vi "Convert Excel to NI Cluster.vi"(8 "error in":errorcluster, 11 "path":path=path "C:/Users/Blueuser/Desktop/Testing/SampleConfiguration.xlsx") -> (0 "error out":errorcluster, 3 "Chassis Settings":T18 {"Chassis Settings"."Master Chassis"."startTriggerLine" items=["None", "PFI_0", "PFI_1", "PFI_2", "PFI_3", "PFI_4", "PFI_5", "PFI_6", "PFI_7", "PFI_8", "PFI_9", "PFI_10", "PFI_11", "PFI_12", "PFI_13", "PFI_14", "PFI_15", "RTSI_PXI_TRIG_0", "RTSI_PXI_TRIG_1", "RTSI_PXI_TRIG_2", "RTSI_PXI_TRIG_3", "RTSI_PXI_TRIG_4", "RTSI_PXI_TRIG_5", "RTSI_PXI_TRIG_6", "RTSI_PXI_TRIG_7"]; "Chassis Settings"."Master Chassis"."startTrigger" items=["aiStartTrigger", "aoStartTrigger"]; "Chassis Settings"."Master Chassis"."triggerSlope" items=["Falling"=10171, "Rising"=10280]; "Chassis Settings"."Master Chassis"."triggerLine" items=["None", "PFI_0", "PFI_1", "PFI_2", "PFI_3", "PFI_4", "PFI_5", "PFI_6", "PFI_7", "PFI_8", "PFI_9", "PFI_10", "PFI_11", "PFI_12", "PFI_13", "PFI_14", "PFI_15", "RTSI_PXI_TRIG_0", "RTSI_PXI_TRIG_1", "RTSI_PXI_TRIG_2", "RTSI_PXI_TRIG_3", "RTSI_PXI_TRIG_4", "RTSI_PXI_TRIG_5", "RTSI_PXI_TRIG_6", "RTSI_PXI_TRIG_7"]; "Chassis Settings"."Master Chassis"."exportClkToLine" items=["Default_RTSI_PXI_TRIG_0", "PFI_0", "PFI_1", "PFI_2", "PFI_3", "PFI_4", "PFI_5", "PFI_6", "PFI_7", "PFI_8", "PFI_9", "PFI_10", "PFI_11", "PFI_12", "PFI_13", "PFI_14", "PFI_15", "RTSI_PXI_TRIG_0", "RTSI_PXI_TRIG_1", "RTSI_PXI_TRIG_2", "RTSI_PXI_TRIG_3", "RTSI_PXI_TRIG_4", "RTSI_PXI_TRIG_5", "RTSI_PXI_TRIG_6", "RTSI_PXI_TRIG_7"]; "Chassis Settings"."Master Chassis"."exportClk" items=["aiSampleClock", "aoSampleClock"]; "Chassis Settings"."Master Chassis"."activeEdge" items=["Falling"=10171, "Rising"=10280]; "Chassis Settings"."Master Chassis"."clkSrc" items=["Onboard10MHzClock", "PFI_0", "PFI_1", "PFI_2", "PFI_3", "PFI_4", "PFI_5", "PFI_6", "PFI_7", "PFI_8", "PFI_9", "PFI_10", "PFI_11", "PFI_12", "PFI_13", "PFI_14", "PFI_15", "RTSI_PXI_TRIG_0", "RTSI_PXI_TRIG_1", "RTSI_PXI_TRIG_2", "RTSI_PXI_TRIG_3", "RTSI_PXI_TRIG_4", "RTSI_PXI_TRIG_5", "RTSI_PXI_TRIG_6", "RTSI_PXI_TRIG_7"]; "DAQ Boards"."Counter Settings"."Position Measurements"."ZIndexMode" items=["AHighBHigh"=10040, "AHighBLow"=10041, "ALowBHigh"=10042, "ALowBLow"=10043]; "DAQ Boards"."Counter Settings"."Position Measurements"."Decoding" items=["Decoding1X"=10090, "Decoding2X"=10091, "Decoding4X"=10092, "DecodingPulseCounting"=10313]; "DAQ Boards"."Counter Settings"."Count Measurements"."CountDirection" items=["Down"=10124, "Up"=10128, "ExternallyControlled"=10326]; "DAQ Boards"."Counter Settings"."Count Measurements"."Edge" items=["Falling"=10171, "Rising"=10280]; "DAQ Boards"."Counter Settings"."Period Measurements"."Edge" items=["Falling"=10171, "Rising"=10280]; "DAQ Boards"."Counter Settings"."Frequency Measurements"."Edge" items=["Falling"=10171, "Rising"=10280]; "DAQ Boards"."Analog Outputs"."ChannelType" items=["Voltage", "Current"]; "DAQ Boards"."Analog Inputs"."ChannelType" items=["Voltage", "Current"]; "DAQ Boards"."DAQConversionRateOption" items=["Default", "Maximum"]; "DAQ Boards"."InputConfiguration" items=["NRSE"=10078, "RSE"=10083, "Differential"=10106, "Pseudodifferential"=12529, "Default"=-1]; "CAN Boards"."Log Files"."Operation" items=["ContinueLoggingInNewFile", "StopLogging"]; "CAN Boards"."Log Files"."LimitType" items=["Footprint", "Time"]; "CAN Boards"."Log Files"."TriggerType" items=["StartLoggingOnNonZero", "StartLoggingOnZero", "EnableLoggingWhenTriggerIsZero", "EnableLoggingWhenTriggerIsNonZero"]; "CAN Boards"."Log Files"."Filter" items=["LogEntireBusTraffic", "ExcludeFrameIDs", "IncludeFrameIDs"]; "CAN Boards"."Log Files"."DataLoggingFileType" items=["TDMS", "NCL"]; "CAN Boards"."TransmitOrderType" items=["AsSubmitted", "ByIdentifier"]; "CAN Boards"."TransceiverType" items=["HS", "LS", "SW"]; "CAN Boards"."Termination" items=["Off", "On"]; "CAN Boards"."Outgoing Frames"."Phase" items=["Unchanged", "Reset"]; "CAN Boards"."Outgoing Frames"."TriggerType" items=["ChannelValueChange", "TriggerChannelNotZero", "ChannelValueChangeOrTriggerChannelNotZero"]})   [LabVIEW 2019, in "Simple SysDef API.lvlib"]
uses:
  <userlib>/SimpleSysDef/Simple SysDef API.lvlib
  <userlib>/SimpleSysDef/_SubVIs/Edit Chassis_Settings.ctl
  <userlib>/SimpleSysDef/_SubVIs/Add Chassis_DAQ Master Settings.ctl
  <userlib>/SimpleSysDef/_SubVIs/Add Chassis_Type.ctl
  <userlib>/SimpleSysDef/_SubVIs/Add DAQ Hardware_Settings.ctl
  <userlib>/SimpleSysDef/_SubVIs/Add DAQ Hardware_Analog Settings.ctl
  <userlib>/SimpleSysDef/_SubVIs/Add DAQ Hardware_Digital Port Settings.ctl
  <userlib>/SimpleSysDef/_SubVIs/Add DAQ Hardware_Digital Settings.ctl
  <userlib>/SimpleSysDef/_SubVIs/Add Frequency Measurement Channels_Settings.ctl
  <userlib>/SimpleSysDef/_SubVIs/Add Count Measurement Channels_Settings.ctl
  NationalInstruments.VeriStand.SystemDefinitionAPI
  <userlib>/SimpleSysDef/_SubVIs/Add Position Measurement Channels_Settings.ctl
  <userlib>/SimpleSysDef/_SubVIs/Add FPGA Hardware_Settings.ctl
  <userlib>/SimpleSysDef/_SubVIs/Add NI-XNET CAN Hardware_Port Settings.ctl
  <userlib>/SimpleSysDef/_SubVIs/Add NI-XNET CAN Hardware_Periodic Frame Settings.ctl
  <userlib>/SimpleSysDef/_SubVIs/Add NI-XNET CAN Hardware_Frame Settings.ctl
  <userlib>/SimpleSysDef/_SubVIs/Add NI-XNET CAN Hardware_Signal Settings.ctl
  <userlib>/SimpleSysDef/_SubVIs/Add NI-XNET CAN Hardware_Sporadic Frame Settings.ctl
  <userlib>/SimpleSysDef/_SubVIs/Add NI-XNET CAN Hardware_Add Log File_Settings.ctl
  <vilib>/Utility/error.llb/Trim Whitespace One-Sided.vi
  <vilib>/regexp/Match Regular Expression.xnode
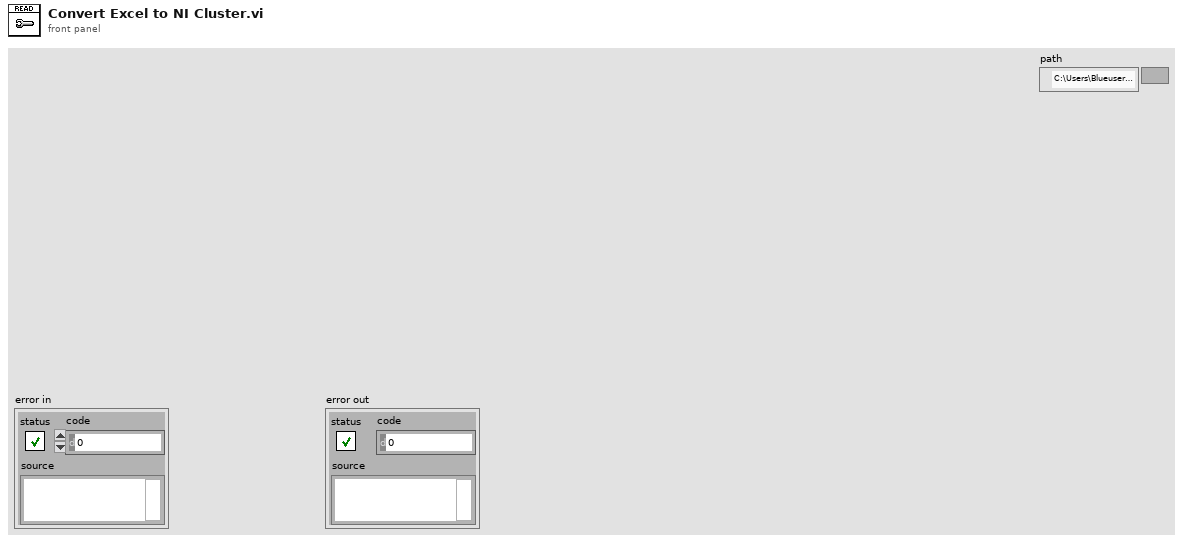
[diagram p1: front panel]
types:
  T1 = typedef "Simple SysDef API.lvlib/Edit Chassis_Settings.ctl" = cluster{"Name":string, "Master Chassis":T2}
  T2 = typedef "Simple SysDef API.lvlib/Add Chassis_DAQ Master Settings.ctl" = cluster{"Type":T3, "DAQ Name":string, "clkSrc":i32, "activeEdge":i32, "exportClk":i32, "exportClkToLine":i32, "triggerLine":i32, "triggerSlope":i32, "startTrigger":i32, "startTriggerLine":i32}
  T3 = typedef "Simple SysDef API.lvlib/Add Chassis_Type.ctl" = enum16{"None", "DAQ", "FPGA", "Timing and Sync", "Automatic"}
  T4 = typedef "Simple SysDef API.lvlib/Add DAQ Hardware_Settings.ctl" = cluster{"Name":string, "Description":string, "InputConfiguration":i32, "TurnOffHWTimedSinglePointAI":bool, "TurnOffHWTimedSinglePointAO":bool, "DAQConversionRateOption":i32, "PortWidth":u16, "Analog Inputs":T5[], "Analog Outputs":T5[], "DIO Port Settings":T6[], "Counter Settings":cluster{"Frequency Measurements":T8[], "Period Measurements":T8[], "Count Measurements":T9[], "Position Measurements":T10[]}}
  T5 = typedef "Simple SysDef API.lvlib/Add DAQ Hardware_Analog Settings.ctl" = cluster{"Name":string, "Units":string, "InitialValue":dbl, "HighLevel":dbl, "LowLevel":dbl, "Channel":u32, "ChannelType":i32, "Alias Name":string}
  T6 = typedef "Simple SysDef API.lvlib/Add DAQ Hardware_Digital Port Settings.ctl" = cluster{"portNumber":u32, "Inverted":bool, "Digital Inputs":T7[], "Digital Outputs":T7[]}
  T7 = typedef "Simple SysDef API.lvlib/Add DAQ Hardware_Digital Settings.ctl" = cluster{"Name":string, "InitialValue":bool, "DigitalLine":u32, "Alias Name":string}
  T8 = typedef "Simple SysDef API.lvlib/Add Frequency Measurement Channels_Settings.ctl" = cluster{"Name":string, "Description":string, "Units":string, "Counter":u32, "DefaultValue":dbl, "Maximum":dbl, "Minimum":dbl, "Edge":i32, "Alias Name":string}
  T9 = typedef "Simple SysDef API.lvlib/Add Count Measurement Channels_Settings.ctl" = cluster{"Name":string, "Description":string, "Units":string, "Counter":u32, "DefaultValue":dbl, "CountDirection":i32, "Edge":i32, "ResetVariable":refnum<k24>, "Alias Name":string}
  T10 = typedef "Simple SysDef API.lvlib/Add Position Measurement Channels_Settings.ctl" = cluster{"Name":string, "Description":string, "Units":string, "Counter":u32, "DefaultValue":dbl, "Decoding":i32, "ZIndexMode":i32, "Alias Name":string}
  T11 = typedef "Simple SysDef API.lvlib/Add FPGA Hardware_Settings.ctl" = cluster{"Path":path, "RIO Name":string, "Aliases":cluster{"Relative Node Path":string, "Alias Name":string}[]}
  T12 = typedef "Simple SysDef API.lvlib/Add NI-XNET CAN Hardware_Port Settings.ctl" = cluster{"Name":string, "Database Name":string, "PortNumber":u16, "ClusterName":string, "BaudRate":u32, "InlineIncoming":bool, "IncomingRate":u32, "InlineOutgoing":bool, "OutgoingRate":u32, "Termination":i32, "Echo":bool, "InputStreamQueueSize":u32, "CANBusOff":bool, "CANBusOffRate":u32, "TransceiverType":i32, "TransmitOrderType":i32, "Cyclic Frames":T13[], "Outgoing Frames":T16[], "Incoming Frames":T14[], "Log Files":T17[]}
  T13 = typedef "Simple SysDef API.lvlib/Add NI-XNET CAN Hardware_Periodic Frame Settings.ctl" = cluster{"Frame Settings":T14, "Trigger Node Path":string, "TriggerType":i32, "Disable Node Path":string}
  T14 = typedef "Simple SysDef API.lvlib/Add NI-XNET CAN Hardware_Frame Settings.ctl" = cluster{"Name":string, "ID":u32, "PayloadLength":u32, "StartTimeOffset":dbl, "Enable64Bit":bool, "Signals":T15[]}
  T15 = typedef "Simple SysDef API.lvlib/Add NI-XNET CAN Hardware_Signal Settings.ctl" = cluster{"Name":string, "Description":string, "Units":string, "DefaultValue":dbl, "Alias Name":string}
  T16 = typedef "Simple SysDef API.lvlib/Add NI-XNET CAN Hardware_Sporadic Frame Settings.ctl" = cluster{"Frame Settings":T14, "Trigger Node Path":string, "TriggerType":i32, "Disable Node Path":string, "EnableSoftwareCyclicTrigger":bool, "TransmitTime":dbl, "Phase":i32}
  T17 = typedef "Simple SysDef API.lvlib/Add NI-XNET CAN Hardware_Add Log File_Settings.ctl" = cluster{"Name":string, "Filename":string, "Destination Folder":path, "NumberOfBytesToRead":u32, "DataLoggingFileType":i32, "TDMSGroupName":string, "TDMSChannelName":string, "Filter":i32, "FrameIDs":string[], "TriggerType":i32, "LimitType":i32, "LimitValue":u32, "Operation":i32, "Retriggerable":bool, "Trigger Node Path":string}
  T18 = cluster{"Chassis Settings":T1, "DAQ Boards":T4[], "FPGA Boards":T11[], "CAN Boards":T12[]}
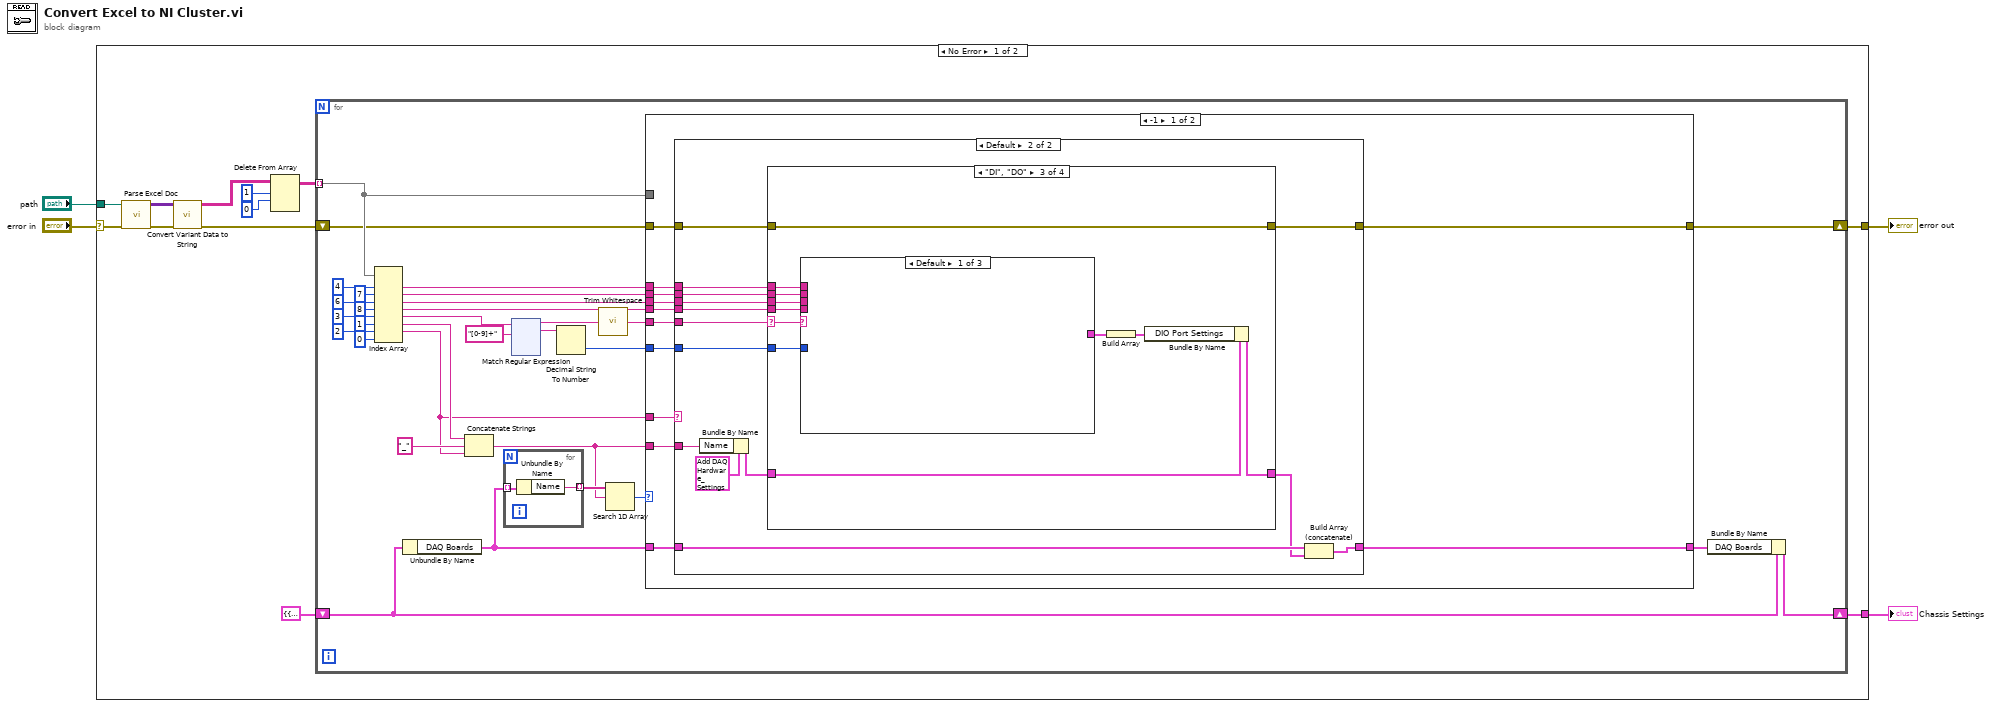
[diagram p0: block diagram]
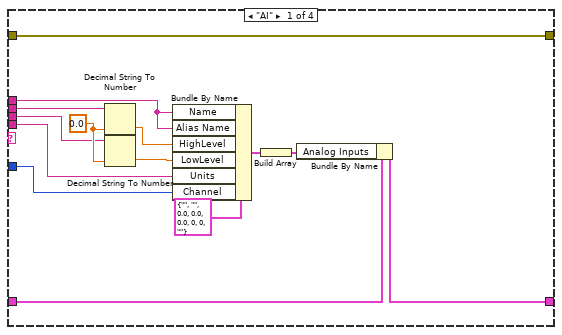
[diagram p3: hidden frame]
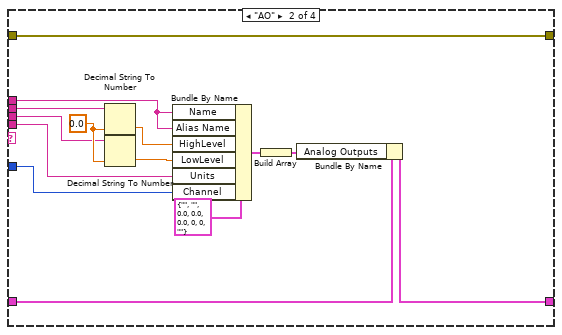
[diagram p4: hidden frame]
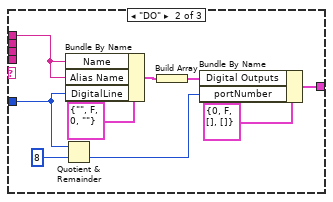
[diagram p5: hidden frame]
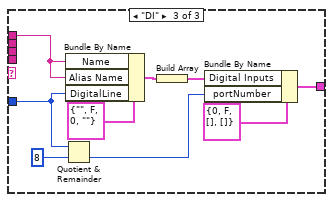
[diagram p6: hidden frame]
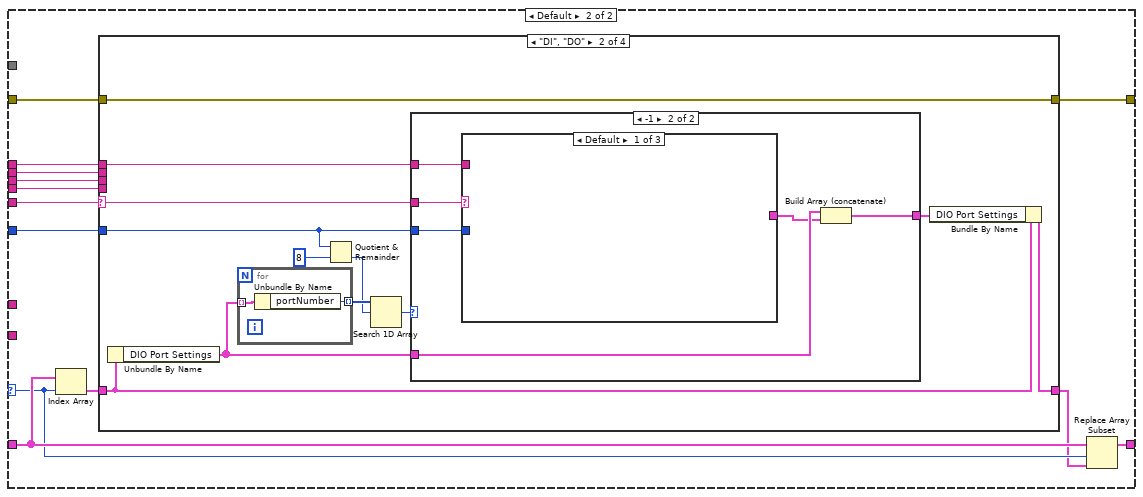
[diagram p8: hidden frame]
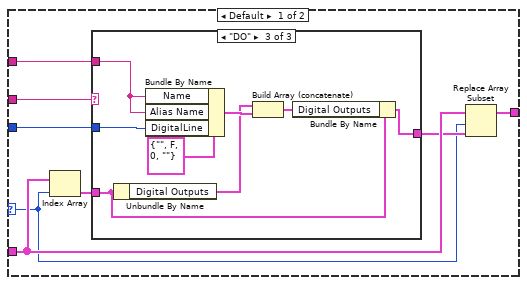
[diagram p10: hidden frame]
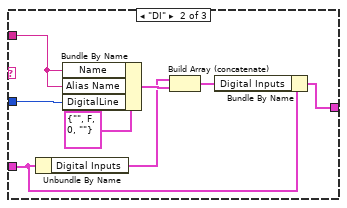
[diagram p12: hidden frame]
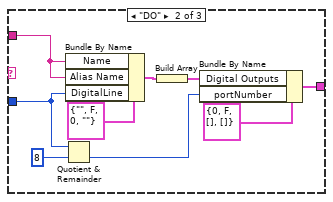
[diagram p13: hidden frame]
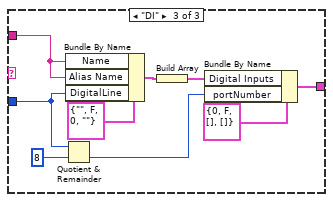
[diagram p14: hidden frame]
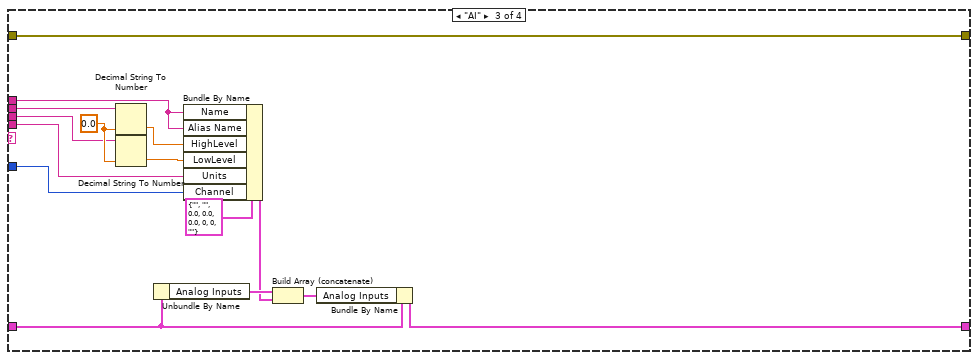
[diagram p15: hidden frame]
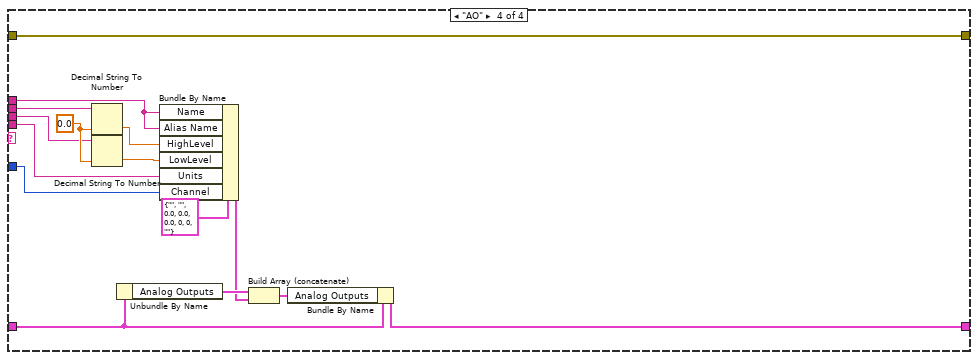
[diagram p16: hidden frame]
diagram:
  n1 = case shown="No Error" "error in" {
    selector: "error in" -> [w13 w361]
    tunnel: "path" -> [w12 _]
    tunnel: [w16 w361] -> w4
    tunnel: [w5 _] -> w1
    frame No Error {
      n2 = call <userlib>:"Parse Excel Doc.vi"("error in (no error)"=w13, "path"=w12) -> ("error out"=w14:errorcluster, "Data"=w15:variant[][])  [unwired: 8 in]
      n3 = call <userlib>:"Convert Variant Data to String.vi"("error in"=w14, "Data"=w15) -> ("error out"=w11:errorcluster, "Data"=w10:string[][])  [unwired: 8 in]
      n4 = Delete From Array(array=w10, length=1, index (row)=0) -> (array with subset deleted=w7:string[][])  [unwired: 1 in, 1 out]
      n5 = for {
        tunnel: w7 -> [w39] mode=indexing
        shift-right: [w37] -> w16
        shift-left: w11 -> [w36]
        shift-right: [w17] -> w5
        shift-left: T18 {"Chassis Settings"={"Name"="Chassis", "Master Chassis"={"Type"=enum."None", "DAQ Name"="", "clkSrc"=0, "activeEdge"=10280, "exportClk"=0, "exportClkToLine"=0, "triggerLine"=0, "triggerSlope"=10280, "startTrigger"=0, "startTriggerLine"=0}}, "DAQ Boards"=[], "FPGA Boards"=[], "CAN Boards"=[]} ("Chassis Settings") -> [w18]
        n6 = Index Array(array=w39, index #1=4 ("index"), index #2=7 ("index"), index #3=6 ("index"), index #4=8 ("index"), index #5=3 ("index"), index #6=1 ("index"), index #7=2 ("index"), index #8=0 ("index")) -> (element #1=w30:string, element #2=w28:string, element #3=w29:string, element #4=w20:string, element #5=w26:string, element #6=w27:string, element #7=w19:string)  [unwired: 1 out]
        n7 = Unbundle By Name(w18) -> ("DAQ Boards"=w41:T4[])
        n8 = Concatenate Strings(w27, "_" ("string"), w19) -> (w33:string)
        n9 = for {
          tunnel: w41 -> [w49] mode=indexing
          tunnel: [w48] -> w43 mode=indexing
          n10 = Unbundle By Name(w49) -> ("Name"=w48:string)
        }
        n11 = xnode "Match Regular Expression"("input string"=w26, "regular expression"="[0-9]+") -> ("before match"=w32:string, "whole match"=w44:string)  [unwired: 4 in, 3 out]
        n12 = Decimal String To Number(string=w44) -> (number=w38:i32)  [unwired: 2 in, 1 out]
        n13 = call <vilib>:"Trim Whitespace.vi"("string"=w32) -> ("trimmed string"=w31:string)  [unwired: 1 in]
        n14 = Search 1D Array(1D array=w43, element=w33) -> (index of element=w42:i32)  [unwired: 1 in]
        n15 = case shown="-1" w42 {
          selector: w42 -> [_ w147]
          tunnel: w41 -> [w61 w149]
          tunnel: [w60 w148] -> w40
          tunnel: w39 -> [_ _]
          tunnel: w36 -> [w57 w142]
          tunnel: w38 -> [w55 w140]
          tunnel: [w58 w143] -> w37
          tunnel: w33 -> [w51 _]
          tunnel: w31 -> [w59 w146]
          tunnel: w30 -> [w56 w141]
          tunnel: w28 -> [w54 w137]
          tunnel: w29 -> [w53 w138]
          tunnel: w20 -> [w52 w139]
          tunnel: w19 -> [w50 _]
          frame -1 {
            n16 = case shown="Default" w50 {
              tunnel: w61 -> [w62 w77]
              tunnel: [w62 w76] -> w60
              tunnel: w59 -> [_ w75]
              tunnel: [w63 w74] -> w58
              tunnel: w57 -> [w63 w73]
              tunnel: w56 -> [_ w71]
              tunnel: w55 -> [_ w70]
              tunnel: w54 -> [_ w69]
              tunnel: w53 -> [_ w68]
              tunnel: w52 -> [_ w67]
              tunnel: w51 -> [_ w65]
              frame "" {
              }
              frame Default {
                n17 = Bundle By Name(cluster=T4 {"Name"="", "Description"="", "InputConfiguration"=10106, "TurnOffHWTimedSinglePointAI"=FALSE, "TurnOffHWTimedSinglePointAO"=FALSE, "DAQConversionRateOption"=0, "PortWidth"=8, "Analog Inputs"=[], "Analog Outputs"=[], "DIO Port Settings"=[], "Counter Settings"={"Frequency Measurements"=[], "Period Measurements"=[], "Count Measurements"=[], "Position Measurements"=[]}} ("DAQ Settings"), "Name"=w65) -> (w72:T4)
                n18 = case shown="\"DI\", \"DO\"" w75 {
                  selector: w75 -> [_ _ w108 _]
                  tunnel: [w91 w105 w116 w136] -> w74
                  tunnel: w73 -> [w91 w105 w116 w136]
                  tunnel: w72 -> [w90 w104 w115 w135]
                  tunnel: w71 -> [w88 w103 w114 _]
                  tunnel: w70 -> [w79 w94 w110 _]
                  tunnel: w69 -> [w85 w100 w113 _]
                  tunnel: w68 -> [w81 w96 w112 _]
                  tunnel: w67 -> [w78 w93 w109 _]
                  tunnel: [w80 w95 w111 w135] -> w66
                  frame "AI" {
                    w83 = 0.0
                    n19 = Decimal String To Number(string=w85, default (0L)=w83) -> (number=w84:dbl)  [unwired: 1 in, 1 out]
                    n20 = Decimal String To Number(string=w81, default (0L)=w83) -> (number=w82:dbl)  [unwired: 1 in, 1 out]
                    n21 = Bundle By Name(cluster=T5 {"Name"="", "Units"="", "InitialValue"=0.0, "HighLevel"=0.0, "LowLevel"=0.0, "Channel"=0, "ChannelType"=0, "Alias Name"=""} ("Analog Input"), "Name"=w88, "Alias Name"=w88, "HighLevel"=w84, "LowLevel"=w82, "Units"=w78, "Channel"=w79) -> (w87:T5)
                    n22 = Build Array(w87) -> (w86:T5[])
                    n23 = Bundle By Name(cluster=w90, "Analog Inputs"=w86) -> (w80:T4)
                  }
                  frame "AO" {
                    w98 = 0.0
                    n24 = Decimal String To Number(string=w100, default (0L)=w98) -> (number=w99:dbl)  [unwired: 1 in, 1 out]
                    n25 = Decimal String To Number(string=w96, default (0L)=w98) -> (number=w97:dbl)  [unwired: 1 in, 1 out]
                    n26 = Bundle By Name(cluster=T5 {"Name"="", "Units"="", "InitialValue"=0.0, "HighLevel"=0.0, "LowLevel"=0.0, "Channel"=0, "ChannelType"=0, "Alias Name"=""} ("Analog Input"), "Name"=w103, "Alias Name"=w103, "HighLevel"=w99, "LowLevel"=w97, "Units"=w93, "Channel"=w94) -> (w102:T5)
                    n27 = Build Array(w102) -> (w101:T5[])
                    n28 = Bundle By Name(cluster=w104, "Analog Outputs"=w101) -> (w95:T4)
                  }
                  frame "DI", "DO" {
                    n29 = case shown="Default" w108 {
                      tunnel: w114 -> [_ w125 w134]
                      tunnel: w113 -> [_ _ _]
                      tunnel: w112 -> [_ _ _]
                      tunnel: w110 -> [_ w119 w128]
                      tunnel: w109 -> [_ _ _]
                      tunnel: [_ w121 w130] -> w107
                      frame Default {
                      }
                      frame "DO" {
                        n30 = Quotient & Remainder(x=w119, y=8) -> (floor(x/y)=w117:i32)  [unwired: 1 out]
                        n31 = Bundle By Name(cluster=T7 {"Name"="", "InitialValue"=FALSE, "DigitalLine"=0, "Alias Name"=""} ("Digital Output"), "Name"=w125, "Alias Name"=w125, "DigitalLine"=w119) -> (w122:T7)
                        n32 = Build Array(w122) -> (w120:T7[])
                        n33 = Bundle By Name(cluster=T6 {"portNumber"=0, "Inverted"=FALSE, "Digital Inputs"=[], "Digital Outputs"=[]} ("DIO Port Settings"), "Digital Outputs"=w120, "portNumber"=w117) -> (w121:T6)
                      }
                      frame "DI" {
                        n34 = Quotient & Remainder(x=w128, y=8) -> (floor(x/y)=w126:i32)  [unwired: 1 out]
                        n35 = Bundle By Name(cluster=T7 {"Name"="", "InitialValue"=FALSE, "DigitalLine"=0, "Alias Name"=""} ("Digital Output"), "Name"=w134, "Alias Name"=w134, "DigitalLine"=w128) -> (w131:T7)
                        n36 = Build Array(w131) -> (w129:T7[])
                        n37 = Bundle By Name(cluster=T6 {"portNumber"=0, "Inverted"=FALSE, "Digital Inputs"=[], "Digital Outputs"=[]} ("DIO Port Settings"), "Digital Inputs"=w129, "portNumber"=w126) -> (w130:T6)
                      }
                    }
                    n38 = Build Array(w107) -> (w106:T6[])
                    n39 = Bundle By Name(cluster=w115, "DIO Port Settings"=w106) -> (w111:T4)
                  }
                  frame Default {
                  }
                }
                n40 = Build Array (concatenate)(w77, w66) -> (w76:T4[])
              }
            }
          }
          frame Default {
            n41 = Index Array(array=w149, index=w147) -> (element=w144:T4)
            n42 = case shown="\"DI\", \"DO\"" w146 {
              selector: w146 -> [_ w160 _ _]
              tunnel: [w150 w152 w227 w242] -> w145
              tunnel: w144 -> [w150 w153 w214 w229]
              tunnel: [w151 w163 w228 w243] -> w143
              tunnel: w142 -> [w151 w163 w228 w243]
              tunnel: w141 -> [_ w161 w220 w235]
              tunnel: w140 -> [_ w158 w216 w231]
              tunnel: w139 -> [_ _ w217 w232]
              tunnel: w138 -> [_ _ w218 w233]
              tunnel: w137 -> [_ _ w219 w234]
              frame Default {
              }
              frame "DI", "DO" {
                n43 = Unbundle By Name(w153) -> ("DIO Port Settings"=w154:T6[])
                n44 = for {
                  tunnel: w154 -> [w213] mode=indexing
                  tunnel: [w212] -> w157 mode=indexing
                  n45 = Unbundle By Name(w213) -> ("portNumber"=w212:u32)
                }
                n46 = Quotient & Remainder(x=w158, y=8) -> (floor(x/y)=w156:i32)  [unwired: 1 out]
                n47 = Search 1D Array(1D array=w157, element=w156) -> (index of element=w155:i32)  [unwired: 1 in]
                n48 = case shown="-1" w155 {
                  selector: w155 -> [w164 _]
                  tunnel: [w165 w192] -> w162
                  tunnel: w161 -> [w171 w189]
                  tunnel: w160 -> [w170 w190]
                  tunnel: w158 -> [w169 w191]
                  tunnel: w154 -> [w167 w193]
                  frame Default {
                    n49 = Index Array(array=w167, index=w164) -> (element=w168:T6)
                    n50 = case shown="\"DO\"" w170 {
                      tunnel: w171 -> [_ w179 w187]
                      tunnel: w169 -> [_ w175 w183]
                      tunnel: [_ w172 w180] -> w166
                      tunnel: w168 -> [_ w173 w181]
                      frame Default {
                      }
                      frame "DI" {
                        n51 = Unbundle By Name(w173) -> ("Digital Inputs"=w174:T7[])
                        n52 = Bundle By Name(cluster=T7 {"Name"="", "InitialValue"=FALSE, "DigitalLine"=0, "Alias Name"=""} ("Digital Output"), "Name"=w179, "Alias Name"=w179, "DigitalLine"=w175) -> (w177:T7)
                        n53 = Build Array (concatenate)(w174, w177) -> (w176:T7[])
                        n54 = Bundle By Name(cluster=w173, "Digital Inputs"=w176) -> (w172:T6)
                      }
                      frame "DO" {
                        n55 = Unbundle By Name(w181) -> ("Digital Outputs"=w182:T7[])
                        n56 = Bundle By Name(cluster=T7 {"Name"="", "InitialValue"=FALSE, "DigitalLine"=0, "Alias Name"=""} ("Digital Output"), "Name"=w187, "Alias Name"=w187, "DigitalLine"=w183) -> (w185:T7)
                        n57 = Build Array (concatenate)(w182, w185) -> (w184:T7[])
                        n58 = Bundle By Name(cluster=w181, "Digital Outputs"=w184) -> (w180:T6)
                      }
                    }
                    n59 = Replace Array Subset(array=w167, new element=w166, index=w164) -> (w165:T6[])
                  }
                  frame -1 {
                    n60 = case shown="Default" w190 {
                      tunnel: w189 -> [_ w202 w211]
                      tunnel: w191 -> [_ w196 w205]
                      tunnel: [_ w198 w207] -> w188
                      frame Default {
                      }
                      frame "DO" {
                        n61 = Quotient & Remainder(x=w196, y=8) -> (floor(x/y)=w194:i32)  [unwired: 1 out]
                        n62 = Bundle By Name(cluster=T7 {"Name"="", "InitialValue"=FALSE, "DigitalLine"=0, "Alias Name"=""} ("Digital Output"), "Name"=w202, "Alias Name"=w202, "DigitalLine"=w196) -> (w199:T7)
                        n63 = Build Array(w199) -> (w197:T7[])
                        n64 = Bundle By Name(cluster=T6 {"portNumber"=0, "Inverted"=FALSE, "Digital Inputs"=[], "Digital Outputs"=[]} ("DIO Port Settings"), "Digital Outputs"=w197, "portNumber"=w194) -> (w198:T6)
                      }
                      frame "DI" {
                        n65 = Quotient & Remainder(x=w205, y=8) -> (floor(x/y)=w203:i32)  [unwired: 1 out]
                        n66 = Bundle By Name(cluster=T7 {"Name"="", "InitialValue"=FALSE, "DigitalLine"=0, "Alias Name"=""} ("Digital Output"), "Name"=w211, "Alias Name"=w211, "DigitalLine"=w205) -> (w208:T7)
                        n67 = Build Array(w208) -> (w206:T7[])
                        n68 = Bundle By Name(cluster=T6 {"portNumber"=0, "Inverted"=FALSE, "Digital Inputs"=[], "Digital Outputs"=[]} ("DIO Port Settings"), "Digital Inputs"=w206, "portNumber"=w203) -> (w207:T6)
                      }
                    }
                    n69 = Build Array (concatenate)(w193, w188) -> (w192:T6[])
                  }
                }
                n70 = Bundle By Name(cluster=w153, "DIO Port Settings"=w162) -> (w152:T4)
              }
              frame "AI" {
                w222 = 0.0
                n71 = Decimal String To Number(string=w219, default (0L)=w222) -> (number=w223:dbl)  [unwired: 1 in, 1 out]
                n72 = Decimal String To Number(string=w218, default (0L)=w222) -> (number=w221:dbl)  [unwired: 1 in, 1 out]
                n73 = Unbundle By Name(w214) -> ("Analog Inputs"=w226:T5[])
                n74 = Bundle By Name(cluster=T5 {"Name"="", "Units"="", "InitialValue"=0.0, "HighLevel"=0.0, "LowLevel"=0.0, "Channel"=0, "ChannelType"=0, "Alias Name"=""} ("Analog Input"), "Name"=w220, "Alias Name"=w220, "HighLevel"=w223, "LowLevel"=w221, "Units"=w217, "Channel"=w216) -> (w215:T5)
                n75 = Build Array (concatenate)(w226, w215) -> (w225:T5[])
                n76 = Bundle By Name(cluster=w214, "Analog Inputs"=w225) -> (w227:T4)
              }
              frame "AO" {
                w237 = 0.0
                n77 = Decimal String To Number(string=w234, default (0L)=w237) -> (number=w238:dbl)  [unwired: 1 in, 1 out]
                n78 = Decimal String To Number(string=w233, default (0L)=w237) -> (number=w236:dbl)  [unwired: 1 in, 1 out]
                n79 = Unbundle By Name(w229) -> ("Analog Outputs"=w241:T5[])
                n80 = Bundle By Name(cluster=T5 {"Name"="", "Units"="", "InitialValue"=0.0, "HighLevel"=0.0, "LowLevel"=0.0, "Channel"=0, "ChannelType"=0, "Alias Name"=""} ("Analog Input"), "Name"=w235, "Alias Name"=w235, "HighLevel"=w238, "LowLevel"=w236, "Units"=w232, "Channel"=w231) -> (w230:T5)
                n81 = Build Array (concatenate)(w241, w230) -> (w240:T5[])
                n82 = Bundle By Name(cluster=w229, "Analog Outputs"=w240) -> (w242:T4)
              }
            }
            n83 = Replace Array Subset(array=w149, new element=w145, index=w147) -> (w148:T4[])
          }
        }
        n84 = Bundle By Name(cluster=w18, "DAQ Boards"=w40) -> (w17:T18)
      }
    }
    frame Error {
    }
  }
  "error out" <- w4
  "Chassis Settings" <- w1
